vi "Read Scheduled.vi"(7 "scheduled time":timestamp, 8 "subchannel (0)":i32, 9 "ack id (0)":u32, 10 "channel":T1) -> (0 "last element?":bool, 1 "remaining":i32, 2 "element":T2, 3 "element valid?":bool, 5 "actual time":timestamp)   [LabVIEW 2019, in "MessengerM.lvlib"]
doc: "Reads an element from a Messenger channel at a scheduled time. The endpoint waits if no element is available in the channel at the scheduled time."
uses:
  <resource>/Channels/MessengerM/MessengerM.lvlib
  <resource>/ChannelSupport/_ChannelSupport/_ChannelSupport.lvlib
  <resource>/Channels/MessengerM/))Channel.ctl
  <resource>/Channels/MessengerM/Element.ctl
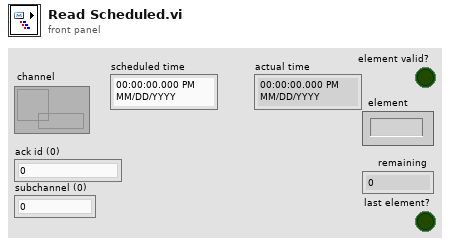
[diagram p1: front panel]
types:
  T1 = typedef "MessengerM.lvlib/))Channel.ctl" = refnum<queue>
  T2 = typedef "MessengerM.lvlib/Element.ctl" = string
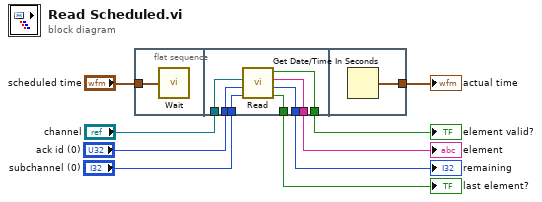
[diagram p0: block diagram]
diagram:
  n1 = flat-sequence {
    tunnel: "scheduled time" -> [w10]
    tunnel: "channel" -> [w17]
    tunnel: [w16] -> w6
    tunnel: [w15] -> w5
    tunnel: "ack id (0)" -> [w14]
    tunnel: "subchannel (0)" -> [w13]
    tunnel: [w12] -> w2
    tunnel: [w11] -> w1
    tunnel: [w18] -> w8
    frame #0 {
      n2 = call <resource>:"Wait.vi"("desired time"=w10) -> ()  [unwired: 2 out]
    }
    frame #1 {
      n3 = call <resource>:"Read.vi"("subchannel (0)"=w13, "ack id (0)"=w14, "channel"=w17) -> ("last element?"=w11:bool, "remaining"=w15:i32, "element"=w16:T2, "element valid?"=w12:bool)  [unwired: 4 in, 1 out]
    }
    frame #2 {
      n4 = Get Date/Time In Seconds() -> (seconds since 1Jan1904=w18:timestamp)
    }
  }
  "element" <- w6
  "actual time" <- w8
  "remaining" <- w5
  "last element?" <- w1
  "element valid?" <- w2
